vi "Mirror_Scan_Pixels_Main_V1.vi"() -> ()   [LabVIEW 2014]
uses:
  Pixel Scan Parameters.ctl
  <vilib>/Analysis/baseanly.llb/Mean (DBL).vi
  <vilib>/Analysis/NI_AALBase.lvlib
panel:
  in  "Set to Zero":bool
  in  "Center Bias":bool
  out "Pixel Map (-1 to 1)":dbl[][](graph)
  in  "Apply Flat":bool
  in  "Start Pixel Scan":bool
  in  "Pixel Scan Parameters":T1={"Scan Start Pixel"=1, "Scan End Pixel"=1, "Pixel Start Value (-1 to 1)"=-0.5, "Pixel End Value (-1 to 1)"=0.5, "Number of Steps"=0.1}
  in  "Exit":bool
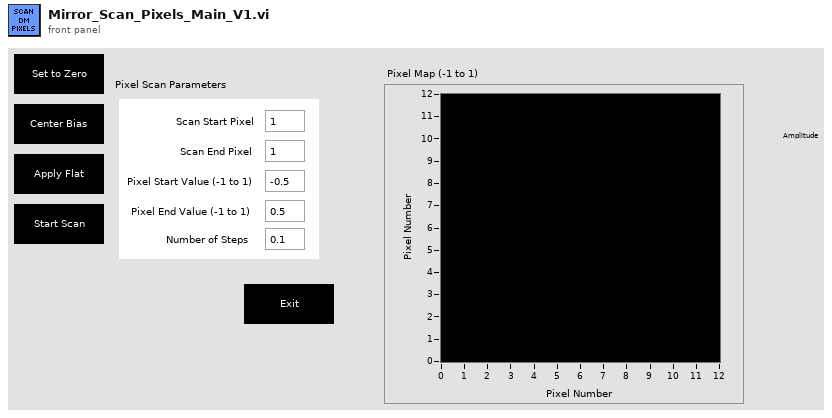
[diagram p1: front panel]
types:
  T1 = typedef "Pixel Scan Parameters.ctl" = cluster{"Scan Start Pixel":i32, "Scan End Pixel":i32, "Pixel Start Value (-1 to 1)":dbl, "Pixel End Value (-1 to 1)":dbl, "Number of Steps":dbl}
  T2 = enum16{"Start Scan", "Reset Counter", "Write DM", "Get Image", "Update Count", "Exit"}
  T3 = enum16{"Reset Counter", "Update Counter", "Get Count"}
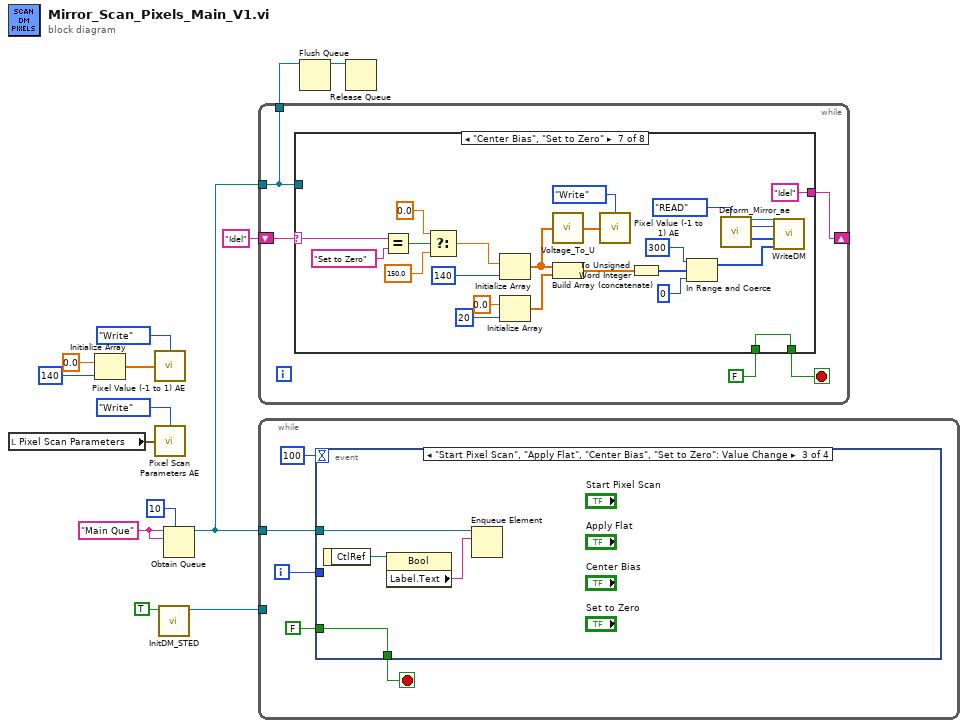
[diagram p0: block diagram]
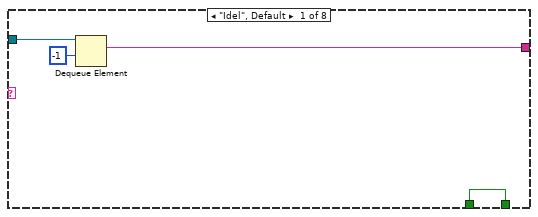
[diagram p2: hidden frame]
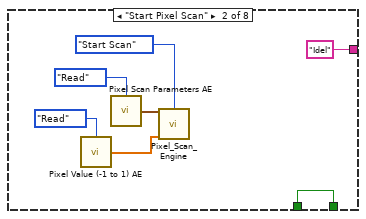
[diagram p3: hidden frame]
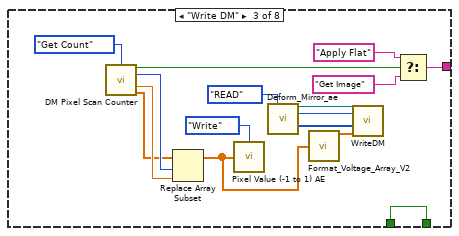
[diagram p4: hidden frame]
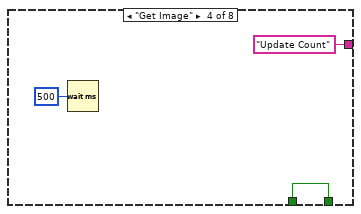
[diagram p5: hidden frame]
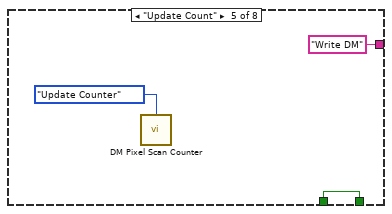
[diagram p6: hidden frame]
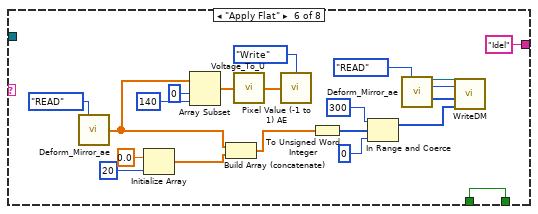
[diagram p7: hidden frame]
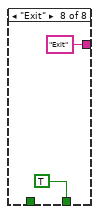
[diagram p8: hidden frame]
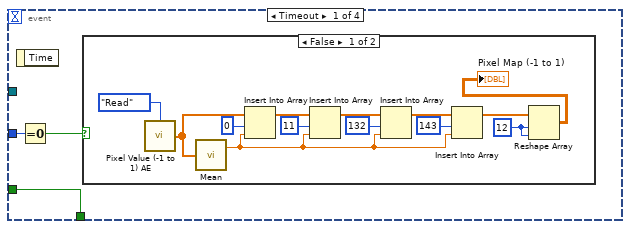
[diagram p9: hidden frame]
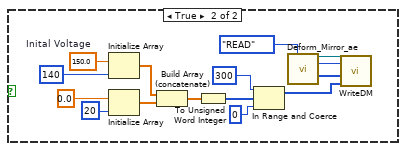
[diagram p10: hidden frame]
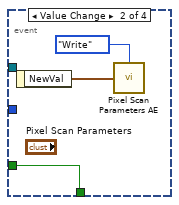
[diagram p11: hidden frame]
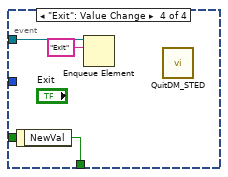
[diagram p12: hidden frame]
diagram:
  w14 = "Main Que" ("name (unnamed)")
  n1 = local read "Pixel Scan Parameters"() -> (w6:T1)
  n2 = Initialize Array(0.0 ("element"), 140 ("dimension size")) -> (w8:dbl[])
  n3 = call "Pixel Value (-1 to 1) AE.vi"("Action"=enum16{"Read", "Write"}."Write", "Pixel Value (-1 to 1)"=w8) -> ()  [unwired: 13 in, 1 out]
  n4 = call "Pixel Scan Parameters AE.vi"("Action"=enum16{"Write", "Read"}."Write", "Pixel Scan Parameters"=w6) -> ()  [unwired: 13 in, 1 out]
  n5 = call "InitDM_STED.vi"("BM Flat"=TRUE) -> ("reference out"=w9:refnum<k7>)  [unwired: 9 in, 1 out]
  n6 = Obtain Queue(max queue size (-1, unlimited)=10, name (unnamed)=w14, element data type=w14) -> (queue out=w12:refnum<queue>)  [unwired: 2 in, 2 out]
  n7 = while {
    tunnel: w12 -> [w15]
    shift-right: [w19] -> _
    shift-left: "Idel" ("name (unnamed)") -> [w18]
    tunnel: [w15] -> w4
    stop <- w17 stop-if-true
    n8 = case shown="\"Center Bias\", \"Set to Zero\"" w18 {
      selector: w18 -> [_ _ _ _ _ _ w79 _]
      tunnel: w15 -> [w23 _ _ _ _ _ _ _]
      tunnel: [w21 "Idel" ("name (unnamed)") w41 "Update Count" ("name (unnamed)") "Write DM" ("name (unnamed)") "Idel" ("name (unnamed)") "Idel" ("name (unnamed)") "Exit" ("name (unnamed)")] -> w19
      tunnel: [w20 w30 w46 w49 w52 w72 w97 TRUE] -> w17
      tunnel: FALSE -> [w20 w30 w46 w49 w52 w72 w97 _]
      frame "Idel", Default {
        n9 = Dequeue Element(queue=w23, timeout in ms (-1)=-1) -> (element=w21:string)  [unwired: 1 in, 3 out]
      }
      frame "Start Pixel Scan" {
        n10 = call "Pixel Value (-1 to 1) AE.vi"("Action"=enum16{"Read", "Write"}."Read") -> ("Pixel Value (-1 to 1) Out"=w26:dbl[])  [unwired: 14 in]
        n11 = call "Pixel Scan Parameters AE.vi"("Action"=enum16{"Write", "Read"}."Read") -> ("Pixel Scan Parameters Out"=w27:T1)  [unwired: 14 in]
        n12 = call "Pixel_Scan_Engine.vi"("Pixel Scan Parameters In"=w27, "Action"=T2."Start Scan", "Initial Pixel Values (-1 to 1)"=w26) -> ()  [unwired: 13 in]
      }
      frame "Write DM" {
        n13 = call "DM Pixel Scan Counter.vi"("Action"=T3."Get Count") -> ("Scan Done"=w44:bool, "DM Pixel"=w32:i32, "Normalized DM Pixel Value"=w34:dbl, "Initial Pixel Values OUT"=w31:dbl[])  [unwired: 11 in]
        n14 = Replace Array Subset(array=w31, new element=w34, index=w32) -> (w33:dbl[])
        n15 = call "Pixel Value (-1 to 1) AE.vi"("Action"=enum16{"Read", "Write"}."Write", "Pixel Value (-1 to 1)"=w33) -> ()  [unwired: 13 in, 1 out]
        n16 = call "Deform_Mirror_ae.vi"("Enum"=enum16{"WRITE", "READ"}."READ") -> ("Refnum Out"=w40:refnum<k7>, "IDs Out"=w39:i32, "Multi Map Data Out"=w38:i32[])  [unwired: 10 in, 2 out]
        n17 = call "Format_Voltage_Array_V2.vi"("Pixel Level (-1 to 1)"=w33) -> ("Voltage Array (Volts)"=w36:dbl[])  [unwired: 13 in, 1 out]
        n18 = call "WriteDM.vi"("reference in"=w40, "nDevId"=w39, "MultiDM  Mapping"=w38, "Voltage Array in"=w36) -> ()  [unwired: 2 in, 2 out]
        n19 = Select(t="Apply Flat" ("name (unnamed)"), s=w44, f="Get Image" ("name (unnamed)")) -> (s? t:f=w41:string)
      }
      frame "Get Image" {
        n20 = Wait (ms)(milliseconds to wait=u32 500) -> ()  [unwired: 1 out]
      }
      frame "Update Count" {
        n21 = call "DM Pixel Scan Counter.vi"("Action"=T3."Update Counter") -> ()  [unwired: 11 in, 4 out]
      }
      frame "Apply Flat" {
        n22 = call "Deform_Mirror_ae.vi"("Enum"=enum16{"WRITE", "READ"}."READ") -> ("Flat Files Out"=w53:dbl[])  [unwired: 10 in, 4 out]
        n23 = Initialize Array(0.0 ("element"), 20 ("dimension size")) -> (w54:dbl[])
        n24 = Array Subset(array=w53, index=0, length=140) -> (w58:dbl[])
        n25 = Build Array (concatenate)(w53, w54) -> (w57:dbl[])
        n26 = call "Voltage_To_U.vi"("Voltages In (Volts)"=w58) -> ("Pixel Value (-1 to 1)"=w61:dbl[])  [unwired: 14 in]
        n27 = call "Pixel Value (-1 to 1) AE.vi"("Action"=enum16{"Read", "Write"}."Write", "Pixel Value (-1 to 1)"=w61) -> ()  [unwired: 13 in, 1 out]
        n28 = To Unsigned Word Integer(number=w57) -> (unsigned 16bit integer=w66:u16[])
        n29 = In Range and Coerce(upper limit=u16 300, x=w66, lower limit=u16 0) -> (coerced(x)=w63:u16[])  [unwired: 1 out]
        n30 = call "Deform_Mirror_ae.vi"("Enum"=enum16{"WRITE", "READ"}."READ") -> ("Refnum Out"=w70:refnum<k7>, "IDs Out"=w69:i32, "Multi Map Data Out"=w68:i32[])  [unwired: 10 in, 2 out]
        n31 = call "WriteDM.vi"("reference in"=w70, "nDevId"=w69, "MultiDM  Mapping"=w68, "Voltage Array in"=w63) -> ()  [unwired: 2 in, 2 out]
      }
      frame "Center Bias", "Set to Zero" {
        n32 = Equal?(x=w79, y="Set to Zero") -> (x = y?=w77:bool)
        n33 = Select(t=0.0 ("element"), s=w77, f=150.0 ("element")) -> (s? t:f=w75:dbl)
        n34 = Initialize Array(w75, 140 ("dimension size")) -> (w95:dbl[])
        n35 = Initialize Array(0.0 ("element"), 20 ("dimension size")) -> (w93:dbl[])
        n36 = call "Voltage_To_U.vi"("Voltages In (Volts)"=w95) -> ("Pixel Value (-1 to 1)"=w80:dbl[])  [unwired: 14 in]
        n37 = Build Array (concatenate)(w95, w93) -> (w94:dbl[])
        n38 = call "Pixel Value (-1 to 1) AE.vi"("Action"=enum16{"Read", "Write"}."Write", "Pixel Value (-1 to 1)"=w80) -> ()  [unwired: 13 in, 1 out]
        n39 = To Unsigned Word Integer(number=w94) -> (unsigned 16bit integer=w85:u16[])
        n40 = In Range and Coerce(upper limit=u16 300, x=w85, lower limit=u16 0) -> (coerced(x)=w82:u16[])  [unwired: 1 out]
        n41 = call "Deform_Mirror_ae.vi"("Enum"=enum16{"WRITE", "READ"}."READ") -> ("Refnum Out"=w89:refnum<k7>, "IDs Out"=w88:i32, "Multi Map Data Out"=w87:i32[])  [unwired: 10 in, 2 out]
        n42 = call "WriteDM.vi"("reference in"=w89, "nDevId"=w88, "MultiDM  Mapping"=w87, "Voltage Array in"=w82) -> ()  [unwired: 2 in, 2 out]
      }
      frame "Exit" {
      }
    }
  }
  n43 = while {
    tunnel: w12 -> [w100]
    tunnel: w9 -> [_]
    i -> [w101]
    stop <- w104 stop-if-true
    n44 = event shown="[2] \"Start Pixel Scan\", \"Apply Flat\", \"Center Bias\", \"Set to Zero\": Value Change" {
      selector: _ -> [_ _ _ _]
      dyn-events: _ -> [_ _ _ _]
      timeout: 100 -> [_ _ _ _]
      tunnel: [w107 w138 w142 w145] -> w104
      tunnel: FALSE -> [w107 w138 w142 _]
      tunnel: w101 -> [w106 _ _ _]
      tunnel: w100 -> [_ _ w141 w144]
      event Timeout {
        n45 = event-data() -> ()  [unwired: 1 in, 1 out]
        n46 = Equal To 0?(x=w106) -> (x = 0?=w105:bool)
        n47 = case shown="False" w105 {
          frame False {
            w119 = 12 ("dimension size")
            n48 = call "Pixel Value (-1 to 1) AE.vi"("Action"=enum16{"Read", "Write"}."Read") -> ("Pixel Value (-1 to 1) Out"=w120:dbl[])  [unwired: 14 in]
            n49 = call-poly <vilib>:"Mean.vi"("X"=w120) -> ("mean"=w116:dbl)  [unwired: 1 out]
            n50 = Insert Into Array(array=w120, index=0, new element=w116) -> (w111:dbl[])
            n51 = Insert Into Array(array=w111, index=11, new element=w116) -> (w113:dbl[])
            n52 = Insert Into Array(array=w113, index=132, new element=w116) -> (w115:dbl[])
            n53 = Insert Into Array(array=w115, index=143, new element=w116) -> (w108:dbl[])
            n54 = Reshape Array(w108, w119, w119) -> (→"Pixel Map (-1 to 1)":dbl[][])
          }
          frame True {
            w132 = 150.0  # Inital Voltage
            n55 = Initialize Array(w132, 140 ("dimension size")) -> (w135:dbl[])
            n56 = Initialize Array(0.0 ("element"), 20 ("dimension size")) -> (w127:dbl[])
            n57 = Build Array (concatenate)(w135, w127) -> (w125:dbl[])
            n58 = To Unsigned Word Integer(number=w125) -> (unsigned 16bit integer=w124:u16[])
            n59 = In Range and Coerce(upper limit=u16 300, x=w124, lower limit=u16 0) -> (coerced(x)=w121:u16[])  [unwired: 1 out]
            n60 = call "Deform_Mirror_ae.vi"("Enum"=enum16{"WRITE", "READ"}."READ") -> ("Refnum Out"=w131:refnum<k7>, "IDs Out"=w130:i32, "Multi Map Data Out"=w129:i32[])  [unwired: 10 in, 2 out]
            n61 = call "WriteDM.vi"("reference in"=w131, "nDevId"=w130, "MultiDM  Mapping"=w129, "Voltage Array in"=w121) -> ()  [unwired: 2 in, 2 out]
          }
        }
      }
      event Value Change {
        n62 = event-data() -> ("NewVal"=w137:T1)  [unwired: 1 in]
        n63 = call "Pixel Scan Parameters AE.vi"("Action"=enum16{"Write", "Read"}."Write", "Pixel Scan Parameters"=w137) -> ()  [unwired: 13 in, 1 out]
      }
      event "Start Pixel Scan", "Apply Flat", "Center Bias", "Set to Zero": Value Change {
        n64 = event-data() -> ("CtlRef"=w140:refnum<vi>)  [unwired: 1 in]
        n65 = property class="Bool"(reference=w140) -> ("Label.Text"=w139:string)  [unwired: 1 in, 2 out]
        n66 = Enqueue Element(queue=w141, element=w139) -> ()  [unwired: 2 in, 3 out]
      }
      event "Exit": Value Change {
        n67 = event-data() -> ("NewVal"=w145:bool)  [unwired: 1 in]
        n68 = Enqueue Element(queue=w144, element="Exit") -> ()  [unwired: 2 in, 3 out]
        n69 = call "QuitDM_STED.vi"() -> ()  [unwired: 12 in]
      }
    }
  }
  n70 = Flush Queue(queue=w4) -> (queue out=w3:refnum<queue>)  [unwired: 1 in, 2 out]
  n71 = Release Queue(queue=w3) -> ()  [unwired: 2 in, 3 out]
